vi "Set Roll Mode.vi"(11 "en":u32) -> (3 "function return":i32)   [LabVIEW 2021, in "vmmso.lvlib"]
doc: "DLL_API int WINAPI SetRollMode(unsigned int en);"
uses:
  vmmso.lvlib
  vmmso.dll
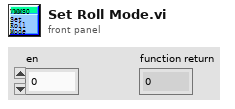
[diagram p1: front panel]
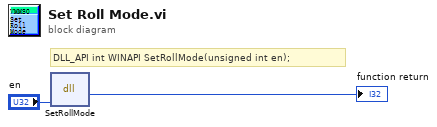
[diagram p0: block diagram]
diagram:
  # "DLL_API int WINAPI SetRollMode(unsigned int en);"
  n1 = dll-call lib="D:/labviewdemo/LabviewDemo 21/vmmso/vmmso.*" fn="SetRollMode"("en"="en") -> (→"function return":i32)  [unwired: 4 in, 2 out]
